vi "Read Mods.vi"(8 "error in (no error)":errorcluster, 11 "ControlMouseDownMsg in":refnum<class "ControlMouseDownMsg.lvclass">) -> (0 "error out":errorcluster, 2 "Mods":cluster{"Double Click":bool, "Menu Key":bool}, 3 "ControlMouseDownMsg out":refnum<class "ControlMouseDownMsg.lvclass">)   [LabVIEW 2015, in "ActorEvents.lvlib" / "ControlMouseDownMsg.lvclass"]
uses:
  ControlMouseDownMsg.lvclass
  ControlMouseDownMsg.lvclass/ControlMouseDownMsg.ctl
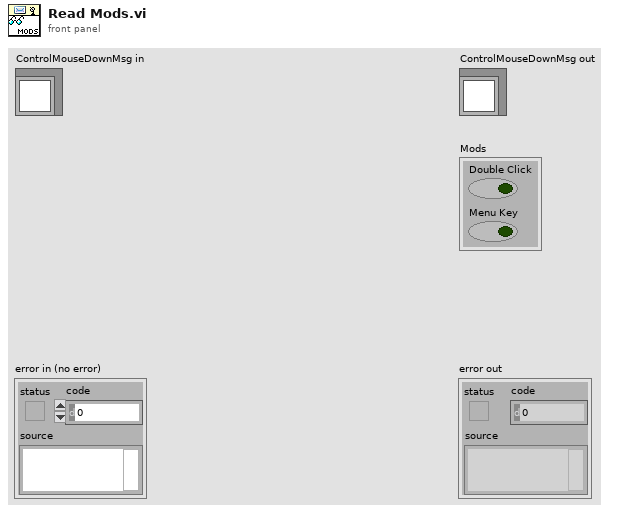
[diagram p1: front panel]
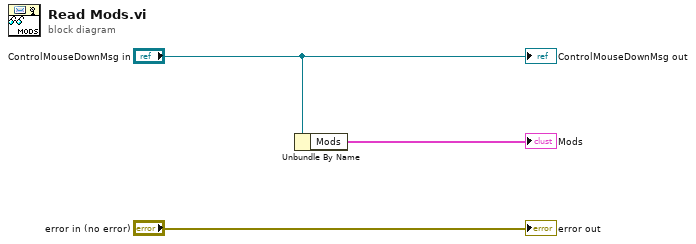
[diagram p0: block diagram]
diagram:
  n1 = Unbundle By Name("ControlMouseDownMsg in") -> ("Mods"=→"Mods":cluster{"Double Click":bool, "Menu Key":bool})
  "error out" <- "error in (no error)"
  "ControlMouseDownMsg out" <- "ControlMouseDownMsg in"
